vi "GetArrayReference.vi"(8 "error in":errorcluster, 11 "Array in":refnum<class "Array.lvclass">) -> (0 "error out":errorcluster, 1 "array reference":refnum<vi>, 3 "Array out":refnum<class "Array.lvclass">)   [LabVIEW 2014, in "Raspberry Pi Compatible Compiler for LabVIEW.lvlib" / "Array.lvclass"]
uses:
  Array.lvclass
  Generic/Generic.lvclass
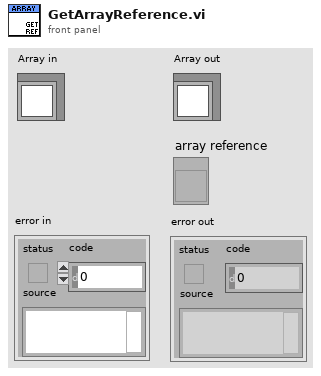
[diagram p1: front panel]
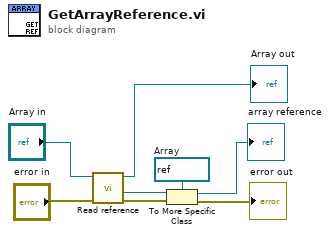
[diagram p0: block diagram]
diagram:
  w6 = refnum<vi> refnum  # Array
  n1 = call "Read reference.vi"("error in"="error in", "GObject in"="Array in") -> ("error out"=w8:errorcluster, "reference"=w7:refnum<vi>, "GObject out"=→"Array out":refnum<class "Array.lvclass">)  [unwired: 5 in]
  n2 = To More Specific Class(target class=w6, reference=w7, error in=w8) -> (specific class reference=→"array reference":refnum<vi>, error out=→"error out":errorcluster)
